vi "SaltedPassword.vi"(10 "HMAC parameters":T1, 11 "Secret":string) -> (1 "Salted password":u8[](array[numeric]))   [LabVIEW 2020, in "wamplv.lvlib" / "WampScramAuthenticator.lvclass"]
uses:
  WampScramAuthenticator.lvclass
  WampScramAuthenticator.lvclass/WampScramAuthenticator.ctl
  HashLib/HashLib.lvclass
  Utils/Utils.lvclass
  TypeDefs/HMAC parameters.ctl
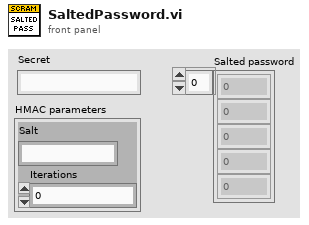
[diagram p1: front panel]
types:
  T1 = typedef "wamplv.lvlib/WampScramAuthenticator.lvclass/HMAC parameters.ctl" = cluster{"Salt":string, "Iterations":i32}
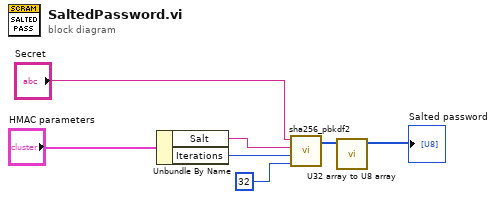
[diagram p0: block diagram]
diagram:
  n1 = Unbundle By Name("HMAC parameters") -> ("Salt"=w4:string, "Iterations"=w3:i32)
  n2 = call "sha256_pbkdf2.vi"("dkLen (32octets=sha256)"=32, "iterations"=w3, "salt"=w4, "password"="Secret") -> ("sha-256"=w1:u32[])  [unwired: 7 in]
  n3 = call "U32 array to U8 array.vi"("Array in"=w1) -> ("Array out"=→"Salted password":u8[])  [unwired: 10 in]
